vi "Automatic_NSEW.vi"() -> ()   [LabVIEW 2010]
panel:
  out "Actual State":enum16{"Off", "N", "E", "S", "W"}(ring)
  in  "?":bool
  in  "Starting State":enum16{"Off", "N", "E", "S", "W"}(ring)
  in  "Interval (ms)":dbl
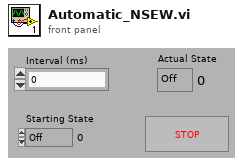
[diagram p1: front panel]
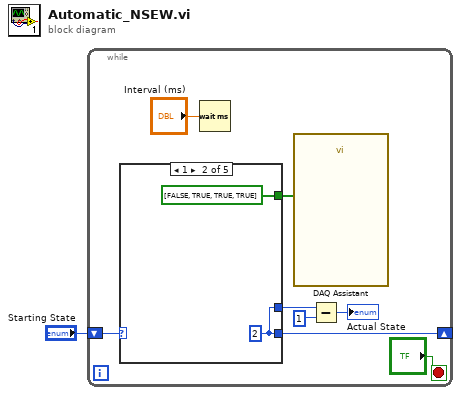
[diagram p0: block diagram]
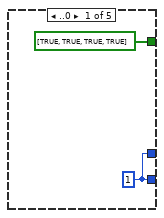
[diagram p2: hidden frame]
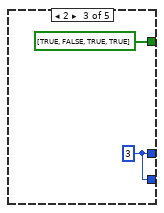
[diagram p3: hidden frame]
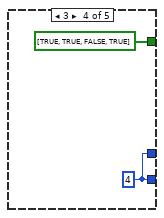
[diagram p4: hidden frame]
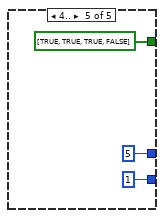
[diagram p5: hidden frame]
diagram:
  n1 = while {
    shift-right: [w7] -> _
    shift-left: "Starting State" -> [w8]
    stop <- "?" stop-if-true
    n2 = case shown="1" w8 {
      tunnel: [bool[] [TRUE, TRUE, TRUE, TRUE] bool[] [FALSE, TRUE, TRUE, TRUE] bool[] [TRUE, FALSE, TRUE, TRUE] bool[] [TRUE, TRUE, FALSE, TRUE] bool[] [TRUE, TRUE, TRUE, FALSE]] -> w5
      tunnel: [w10 w13 w14 w16 1] -> w7
      tunnel: [w10 w13 w14 w16 5] -> w3
      frame ..0 {
        w10 = 1
      }
      frame 1 {
        w13 = 2
      }
      frame 2 {
        w14 = 3
      }
      frame 3 {
        w16 = 4
      }
      frame 4.. {
      }
    }
    n3 = Wait (ms)(milliseconds to wait="Interval (ms)") -> ()  [unwired: 1 out]
    n4 = call "DAQ Assistant"("data"=w5) -> ()  [unwired: 17 in, 2 out]
    n5 = Subtract(x=w3, y=1) -> (x-y=→"Actual State":i32)
  }
